vi "Heater_D2XX.vi"(8 "error in (no error) 2":errorcluster, 11 "Numeric 2":i32) -> (0 "error out 2":errorcluster)   [LabVIEW 2019]
uses:
  D2XX_HeaterStage/D2XX_HeaterStage.lvlib
  <userlib>/LevyLab/Relay Box/D2XX_Functions/D2XX_Functions.lvlib
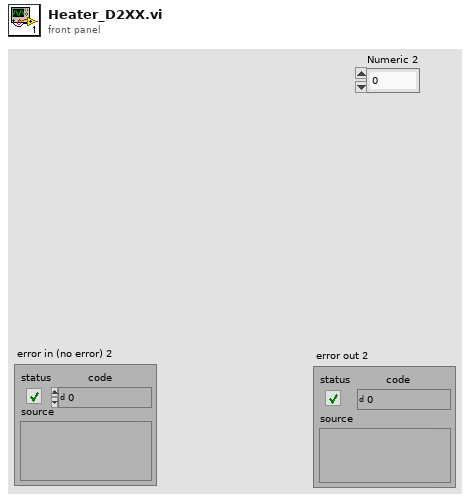
[diagram p1: front panel]
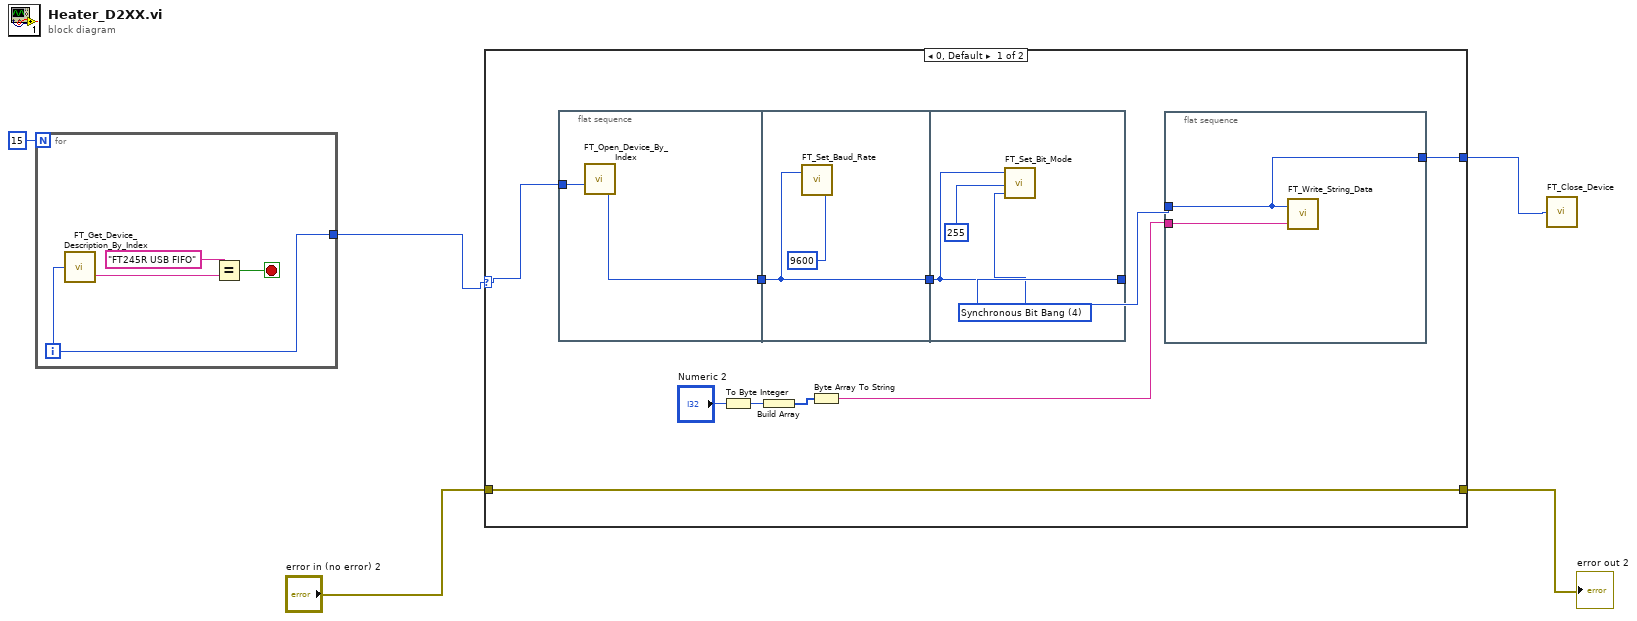
[diagram p0: block diagram]
diagram:
  n1 = for {
    N: 15 -> [_]
    tunnel: [w6] -> w2
    i -> [w6]
    stop <- w7 stop-if-true
    n2 = call "FT_Get_Device_Description_By_Index.vi"("Device Index"=w6) -> ("Device Description"=w8:string)  [unwired: 1 out]
    n3 = Equal?(x="FT245R USB FIFO", y=w8) -> (x = y?=w7:bool)
  }
  n4 = case shown="0, Default" w2 {
    selector: w2 -> [w11 w29]
    tunnel: [w12 w30] -> w3
    tunnel: "error in (no error) 2" -> [w12 w30]
    tunnel: [w10 w29] -> w1
    frame 0, Default {
      n5 = flat-sequence {
        tunnel: w11 -> [w21]
        tunnel: [w20] -> w19
        tunnel: w19 -> [w23]
        tunnel: [w23] -> w18
        tunnel: [w26] -> w14
        tunnel: w18 -> [w26]
        frame #0 {
          n6 = call "FT_Open_Device_By_Index.vi"("Device Index"=w21) -> ("Handle"=w20:u32)  [unwired: 1 out]
        }
        frame #1 {
          n7 = call <userlib>:"FT_Set_Baud_Rate.vi"("Baud Rate"=u32 9600, "Handle"=w23) -> ()  [unwired: 1 out]
        }
        frame #2 {
          w24 = u8 4 items=["Reset Bit Mode"=0, "Asynchronous Bit Bang"=1, "MPSSE"=2, "Synchronous Bit Bang"=4, "MCU Host Bus Emulation"=8, "Fast Opto-Isolated Serial"=16, "CBUS Bit Bang"=32, "Single Channel 245 Synchronous FIFO"=64] ("Bit Mode")
          n8 = call <userlib>:"FT_Set_Bit_Mode.vi"("Bit Mode"=w24, "Bit Mode Mask"=u8 255, "Handle"=w26) -> ()  [unwired: 1 out]
        }
      }
      n9 = To Byte Integer(number="Numeric 2") -> (8bit integer=w17:i8)
      n10 = Build Array(w17) -> (w16:i8[])
      n11 = Byte Array To String(unsigned byte array=w16) -> (string=w15:string)
      n12 = flat-sequence {
        tunnel: w14 -> [w28]
        tunnel: [w28] -> w10
        tunnel: w15 -> [w27]
        frame #0 {
          n13 = call "FT_Write_String_Data.vi"("Buffer"=w27, "Handle"=w28) -> ()  [unwired: 2 out]
        }
      }
    }
    frame 1 {
    }
  }
  "error out 2" <- w3
  n14 = call "FT_Close_Device.vi"("Handle"=w1) -> ()  [unwired: 1 out]
